vi "Format Target Name.vi"(8 "error in":errorcluster, 11 "Sub Obj":refnum<class "Sub Object.lvclass">) -> (0 "error out":errorcluster, 2 "Name":string)   [LabVIEW 2020, in "CANopen.lvlib" / "PDO Mapping.lvclass"]
uses:
  PDO Mapping.lvclass
  PDO Mapping.lvclass/PDO Mapping.ctl
  Sub Object/Sub Object.lvclass
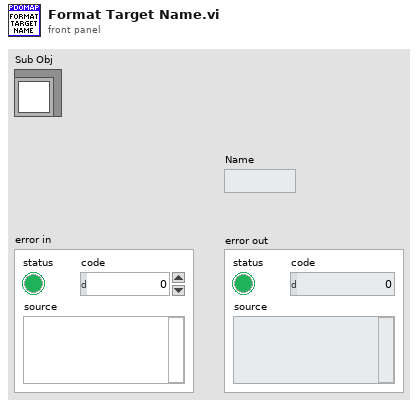
[diagram p1: front panel]
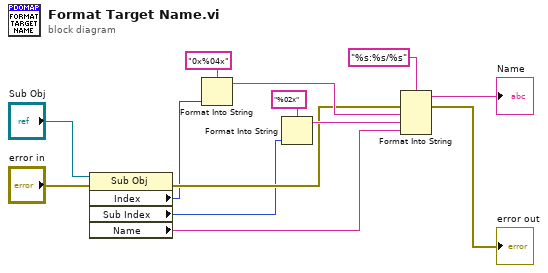
[diagram p0: block diagram]
diagram:
  n1 = property class="Sub Obj"(reference="Sub Obj", error in="error in") -> (error out=w5:errorcluster, "Index"=w3:u16, "Sub Index"=w2:u8, "Name"=w1:string)  [unwired: 1 out]
  n2 = Format Into String(format string="0x%04x", w3) -> (resulting string=w8:string)  [unwired: 2 in, 1 out]
  n3 = Format Into String(format string="%02x", w2) -> (resulting string=w7:string)  [unwired: 2 in, 1 out]
  n4 = Format Into String(format string="%s:%s/%s", error in=w5, w8, w7, w1) -> (resulting string=→"Name":string, error out=→"error out":errorcluster)  [unwired: 1 in]
